vi "LEP_RV_DestroyOpBox.vi"(1 "error in (no error)":errorcluster) -> (0 "error out":errorcluster)   [LabVIEW 2011]
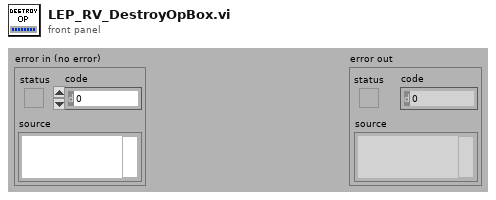
[diagram p1: front panel]
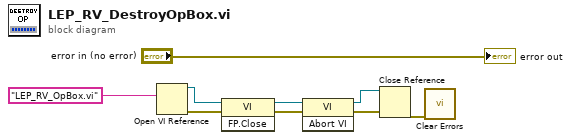
[diagram p0: block diagram]
diagram:
  n1 = Open VI Reference(vi path="LEP_RV_OpBox.vi") -> (vi reference=w7:refnum<vi>, error out=w8:errorcluster)  [unwired: 5 in]
  n2 = invoke class="VI" method="FP.Close"(reference=w7, error in=w8) -> (reference out=w5:refnum<vi>, error out=w6:errorcluster)  [unwired: 1 in, 1 out]
  n3 = invoke class="VI" method="Abort VI"(reference=w5, error in=w6) -> (reference out=w3:refnum<vi>, error out=w4:errorcluster)  [unwired: 1 in, 1 out]
  n4 = Close Reference(reference=w3, error in (no error)=w4) -> (error out=w1:errorcluster)
  n5 = call <vilib>:"Clear Errors.vi"("error in (no error)"=w1) -> ()  [unwired: 6 in, 1 out]
  "error out" <- "error in (no error)"
